vi "DAQ_Analog_Stop.vi"(8 "error in (no error)":errorcluster, 11 "task/channels in":refnum<k21>="Photodetectors") -> (0 "error out":errorcluster)   [LabVIEW 2018]
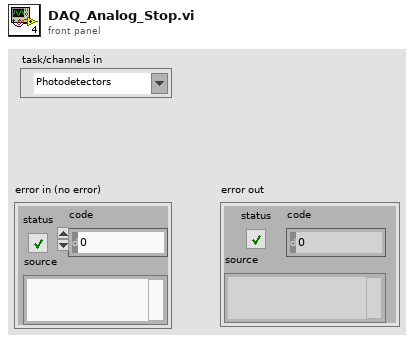
[diagram p1: front panel]
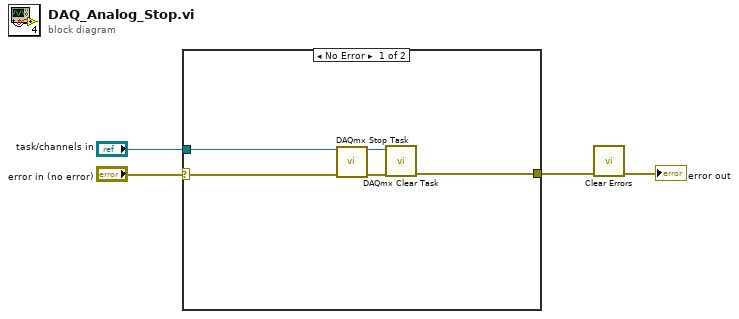
[diagram p0: block diagram]
diagram:
  n1 = case shown="No Error" "error in (no error)" {
    selector: "error in (no error)" -> [w5 w10]
    tunnel: [w7 w10] -> w4
    tunnel: "task/channels in" -> [w6 _]
    frame No Error {
      n2 = call "DAQmx Stop Task.vi"("task/channels in"=w6, "error in"=w5) -> ("task out"=w9:refnum<k21>, "error out"=w8:errorcluster)  [unwired: 12 in]
      n3 = call "DAQmx Clear Task.vi"("task in"=w9, "error in"=w8) -> ("error out"=w7:errorcluster)  [unwired: 13 in]
    }
    frame Error {
    }
  }
  n4 = call "Clear Errors.vi"("error in (no error)"=w4) -> ("error out"=→"error out":errorcluster)  [unwired: 5 in, 1 out]
